vi "Design 2-Band Filter Banks.vi"() -> ()   [LabVIEW 2023]
doc: "This example demonstrates how to use the <b>DFD 2-band QMF Filter Bank Design</b> VI to design a 2-band filter bank.\n\nComplete the following steps to use this VI:\n1) Run this VI.\n2) Observe the <b>Magnitude Response</b> and <b>Phase Response</b> of the lowpass and highpass bands.\n3) Increase the <b>Order</b>. Observe the change in the <b>Magnitude Response</b>. The transition band is sharper.\n4) Change the <b>Roll Off</b>. Observe the change in the <b>Magnitude Response</b>. The larger the <b>Roll Off</b>, the wider the transition band.\n5) Set <b>Phase Option</b> to Linear Phase. Observe the change in the <b>Phase Response</b>. The phase is linear.\n6) Change the <b>Weight</b>. Observe the change in the <b>Magnitude Response</b>. This input is valid only when <b>Phase Option</b> is Linear Phase."
uses:
  <vilib>/addons/Digital Filter Design/_Objects.llb/DFD Phase Setting.ctl
  <vilib>/addons/Digital Filter Design/NI_DigFilter_FilterBank.lvlib
  <vilib>/addons/Digital Filter Design/NI_DigFilterLicensed.lvlib
panel:
  out "Error Message":string
  in  "stop":bool
  out "Phase Response":cluster{"Y":dbl[], "Y":dbl[]}[](graph)
  out "Magnitude Response":cluster{"Y":dbl[], "Y":dbl[]}[](graph)
  in  "Weight":dbl=0.5 min=0.0 max=1.0 step=0.01
  in  "Stopband Attenuation [dB]":dbl=40.0
  in  "Roll Off":dbl=0.2 min=0.01 max=0.99
  in  "Order":i32=31 min=3 max=61 step=2
  in  "Phase Option":u16(ring) items=["Min-Max Phase", "Linear Phase"]
  # "Select Help>>Show Context Help and move the cursor over the VI icon for more information."
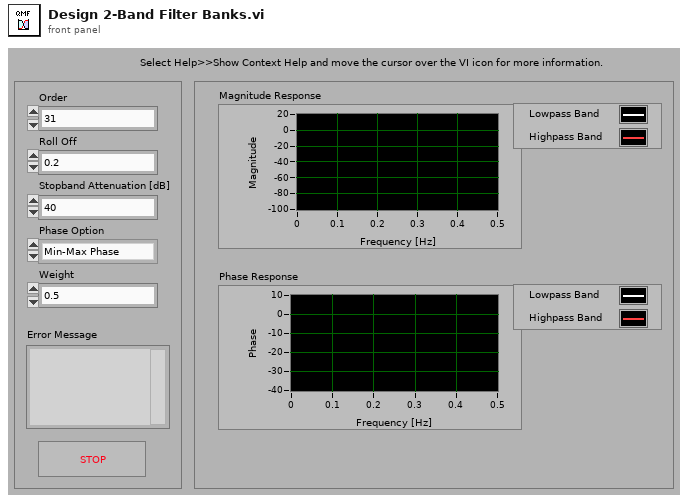
[diagram p1: front panel]
types:
  T1 = typedef "NI_DigFilterLicensed.lvlib/DFD Phase Setting.ctl" = cluster{"unwrap? (F)":bool, "degree? (F)":bool}
  T2 = typedef "NI_DigFilter_FilterBank.lvlib/DFD Filter Bank Obj.ctl" = cluster{"mFBank_AnalysisFilters":T3[], "mFBank_SynthesisFilters":T3[], "mFBank_#Bands":i32, "mFBank_ProcMethod":T8, "mFBank_Coeffs":dbl[], "mFBank_Gain":dbl, "mFBank_Delay":i32, "mFBank_Type":T9}
  T3 = typedef "NI_DigFilterLicensed.lvlib/DFD Multirate Filter Obj.ctl" = cluster{"mMRate_Structure":enum16{"CIC", "FIR", "IIR", "Lattice"}, "mMRate_Mode":T4, "mMRate_Factor":i32, "mMRate_FIRParams":cluster{"mMRate_FIR_H":dbl[], "mMRate_FIR_IsNyquist?":bool, "mMRate_FIR_IsSymmetric?":bool}, "mMRate_CICParams":cluster{"mMRate_CIC_#Stage":i32, "mMRate_CIC_Lag":i32, "mMRate_CIC_Type":enum16{"Lowpass", "Highpass"}}, "mMRate_Order":i32, "mMRate_Version":string, "mMRate_Comments":string, "mMRate_RationalFactor":cluster{"mMRate_L":i32, "mMRate_M":i32}, "mMRate_Fs":dbl, "mMRate_Quantized?":bool, "mMRate_QFilterGain":dbl, "mMRate_CoefWl":i16, "mMRate_Scaling":cluster{"mMRate_ScaleByPowerOf2?":bool, "mMRate_ScaleType":T5}, "mMRate_InputWl":i16, "mMRate_OutputWl":i16, "mMRate_OutputMode":T6, "mMRate_MultMode":T7, "mMRate_BitPruning":bool, "mMRate_GainWl":i16, "mMRate_OutputFwl":i16, "mMRate_SumIwl":i16, "mMRate_InputIwl ":i16, "mMRate_SumWl":i16, "mMRate_CoefIwl":i16}
  T4 = typedef "NI_DigFilterLicensed.lvlib/DFD Multirate Mode.ctl" = i16
  T5 = typedef "NI_DigFilterLicensed.lvlib/DFD Coef Norm Type.ctl" = enum16{"No Norm", "Time Domain 1-Norm", "Time Domain 2-Norm", "Time Domain Inf-Norm"}
  T6 = typedef "NI_DigFilterLicensed.lvlib/DFD Round-off Mode.ctl" = enum16{"Nearest", "Truncation"}
  T7 = typedef "NI_DigFilterLicensed.lvlib/DFD FXP MRate Multiply Mode.ctl" = enum16{"Truncated", "Full"}
  T8 = typedef "NI_DigFilter_FilterBank.lvlib/DFD Filter Bank Processing Method.ctl" = enum16{"General", "2-Band QMF Lattice", "Cosine-Modulated"}
  T9 = typedef "NI_DigFilter_FilterBank.lvlib/DFD Filter Bank Type.ctl" = u16
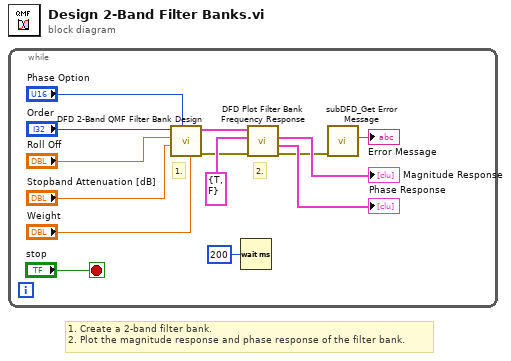
[diagram p0: block diagram]
diagram:
  # "1. Create a 2-band filter bank.\n2. Plot the magnitude response and phase response of the filter bank."
  n1 = while {
    stop <- "stop" stop-if-true
    # "2."
    # "1."
    n2 = call <vilib>:"DFD 2-Band QMF Filter Bank Design.vi"("weight"="Weight", "phase option"="Phase Option", "stopband attenuation [dB]"="Stopband Attenuation [dB]", "roll off"="Roll Off", "order"="Order") -> ("error out"=w5:errorcluster, "filter bank out"=w9:T2)  [unwired: 4 in, 1 out]
    n3 = Wait (ms)(milliseconds to wait=u32 200) -> ()  [unwired: 1 out]
    n4 = call <vilib>:"DFD Plot Filter Bank Frequency Response.vi"("error in (no error)"=w5, "phase view"=T1 {"unwrap? (F)"=TRUE, "degree? (F)"=FALSE}, "filter bank in"=w9) -> ("error out"=w2:errorcluster, "phase responses"=→"Phase Response":cluster{"Y":dbl[], "Y":dbl[]}[], "magnitude responses"=→"Magnitude Response":cluster{"Y":dbl[], "Y":dbl[]}[])  [unwired: 5 in, 1 out]
    n5 = call <vilib>:"subDFD_Get Error Message.vi"("error in (no error)"=w2) -> ("Error Message"=→"Error Message":string)  [unwired: 10 in]
  }
